vi "VFD_No TCHX.vi"() -> (0 "GS1 Communication Error Out":errorcluster)   [LabVIEW 2017]
uses:
  <vilib>/Platform/TimedLoop/XDataNode/timing_clust.ctl
  <vilib>/Platform/TimedLoop/XDataNode/nitl_modes.ctl
  <vilib>/Platform/TimedLoop/XDataNode/wakeup.ctl
  <vilib>/NI Modbus.llb/MB Serial Master Query Write Single Register (poly).vi
  <vilib>/Platform/TimedLoop/XDataNode/XDataNode.xnode
  <vilib>/Platform/TimedLoop/XDataNode/XDNodeRunTimeDep.lvlib
panel:
  in  "GS1 Communication Error In":errorcluster
  out "Iteration Duration":i64
  out "Finished Late? [i-1]":bool
  out "CTAH Initializaton Error":errorcluster
  out "CTAH Initialization Loop Time (ms)":u32
  out "Pump Initializaton Error":errorcluster
  out "Pump Initialization Loop Time (ms)":u32
  # "Troubleshooting Modbus communication using third-party VIs and native I/O Server"
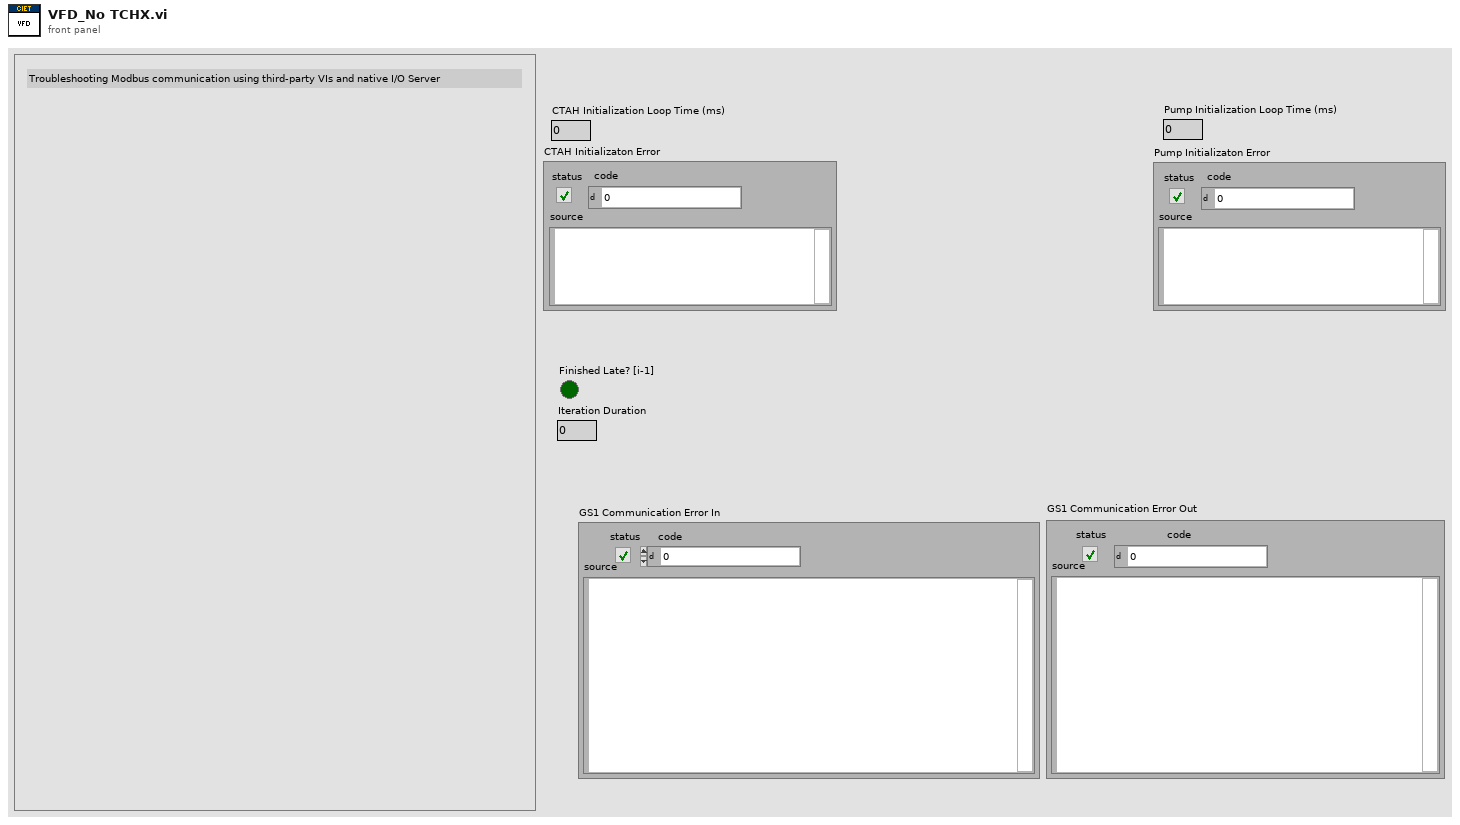
[diagram p1: front panel]
types:
  T1 = cluster{"Mode":enum16{"RTU", "ASCII"}, "Slave Address":u8}
  T2 = typedef "XDNodeRunTimeDep.lvlib/timing_clust.ctl" = cluster{"Expected End [f-1]":u64, "Actual End [f-1]":u64, "Finished Late? [f-1]":bool, "Expected End [i-1]":u64, "Actual End [i-1]":u64, "Finished Late? [i-1]":bool, "Expected Start [i]":u64, "Actual Start [i]":u64, "Expected Start [f]":u64, "Actual Start [f]":u64, "Source Name":string, "Structure Name":string, "Period":i64, "Deadline":i64, "Offset":i64, "Start":i64, "Priority":i32, "Timeout":i32, "Mode":T3, "Wakeup Reason":T4, "Error":errorcluster, "Source Type":string, "Secondary Source Type":string, "Global End Time":u64, "Global Start Time":u64, "Frame Duration":u64, "Iteration Duration":u64, "Assigned CPU":i32, "I/O Scan Engine Mode":u32}
  T3 = typedef "XDNodeRunTimeDep.lvlib/nitl_modes.ctl" = enum32{"No Change", "Process missed periods, maintain original phase", "Discard missed periods, maintain original phase", "Process missed periods, ignore original phase", "Discard missed periods, ignore original phase"}
  T4 = typedef "XDNodeRunTimeDep.lvlib/wakeup.ctl" = enum32{"Normal", "Aborted", "Asynchronous wakeup", "Timing source error", "Timed loop error", "Timeout"}
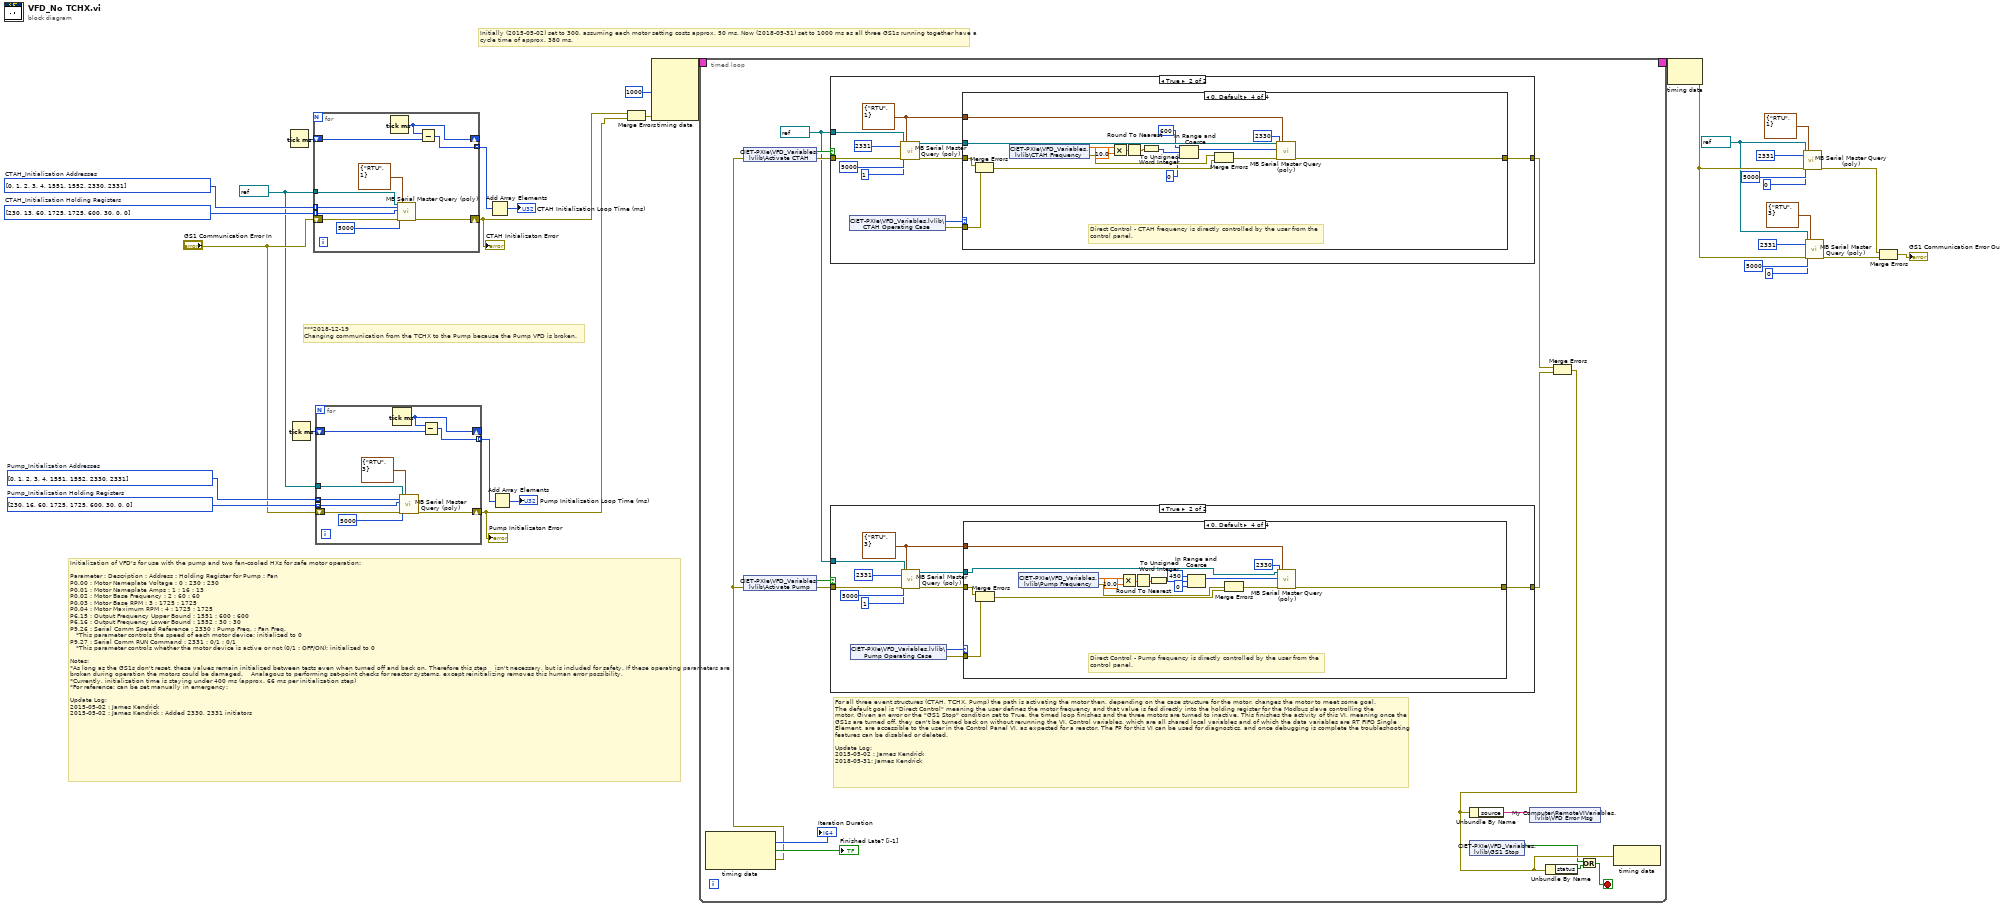
[diagram p0: block diagram]
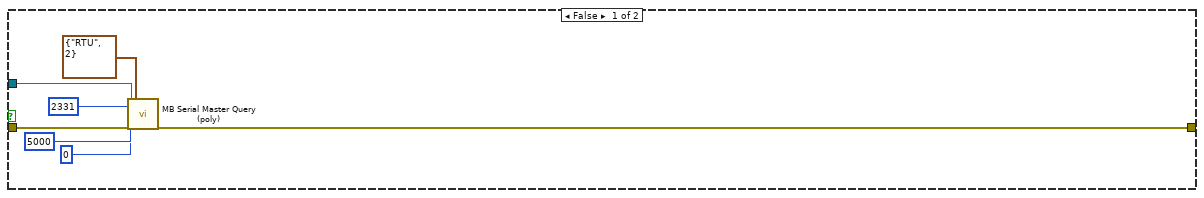
[diagram p2: hidden frame]
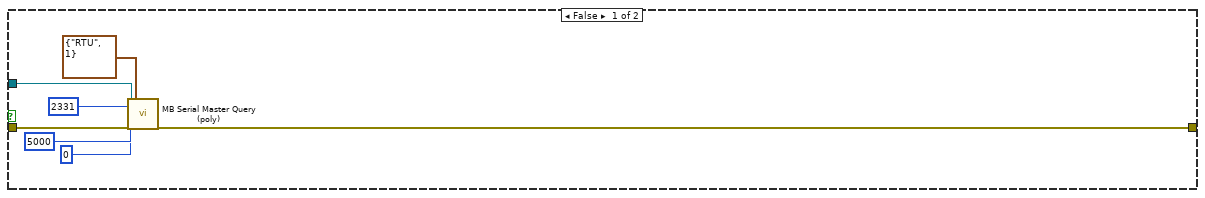
[diagram p6: hidden frame]
diagram:
  w4 = refnum<visa-resource-name> "VFD" ("VISA resource name")
  w5 = refnum<visa-resource-name> "VFD" ("VISA resource name")
  w22 = u16[] [230, 13, 60, 1725, 1725, 600, 30, 0, 0]  # CTAH_Initialization Holding Registers
  w23 = u16[] [0, 1, 2, 3, 4, 1551, 1552, 2330, 2331]  # CTAH_Initialization Addresses
  w30 = u16[] [230, 16, 60, 1725, 1725, 600, 30, 0, 0]  # Pump_Initialization Holding Registers
  w31 = u16[] [0, 1, 2, 3, 4, 1551, 1552, 2330, 2331]  # Pump_Initialization Addresses
  # "***2018-12-19\nChanging communication from the TCHX to the Pump because the Pump VFD is broken."
  # "Initially (2015-05-02) set to 300, assuming each motor setting costs approx. 50 ms. Now (2018-05-31) set to 1000 ms as all three GS1s running together have a \ncycle time of approx. 380 ms."
  # "Initialization of VFD's for use with the pump and two fan-cooled HXs for safe motor operation:\n\nParameter : Description : Address : Holding Register for Pump : Fan\nP0.00 : Motor Nameplate Voltage : 0 : 230 : 230\nP0.01 : Motor Nameplate Amps : 1 : 16 : 13\nP0.02 : Motor Base Frequency : 2 : 60 : 60\nP0.03 : Motor Base RPM : 3 : 1725 : 1725\nP0.04 : Motor Maximum RPM : 4 : 1725 : 1725\nP6.15 : Output Frequency Upper Bound : 1551 : 600 : 600\nP6.16 : Output Frequency Lower Bound : 1552 : 30 : 30\nP9.26 : Serial Comm Speed Reference : 2330 : Pump Freq. : Fan Freq. \n   *This parameter controls the speed of each motor device; initialized to 0\nP9.27 : Serial Comm RUN Command : 2331 : 0/1 : 0/1\n   *This parameter controls whether the motor device is active or not (0/1 : OFF/ON); initialized to 0\n\nNotes:\n*As long as the GS1s don't reset, these values remain initialized between tests even when turned off and back on. Therefore this step    isn't necessary, but is included for safety. If these operating parameters are broken during operation the motors could be damaged.    Analagous to performing set-point checks for reactor systems, except reinitializing removes this human error possibility.\n*Currently, initialization time is staying under 400 ms (approx. 66 ms per initialization step)\n*For reference; can be set manually in emergency:\n\nUpdate Log:\n2015-05-02 : James Kendrick \n2015-05-02 : James Kendrick : Added 2330, 2331 initiators"
  n1 = Tick Count (ms)() -> (millisecond timer value=w21:u32)
  n2 = Tick Count (ms)() -> (millisecond timer value=w29:u32)
  n3 = for {
    shift-right: [w39] -> w10
    shift-left: "GS1 Communication Error In" -> [w40]
    tunnel: w23 -> [w38] mode=indexing
    tunnel: w22 -> [w37] mode=indexing
    shift-right: [w34] -> _
    shift-left: w21 -> [w36]
    tunnel: [w35] -> w20 mode=indexing
    tunnel: w5 -> [w33]
    n4 = Tick Count (ms)() -> (millisecond timer value=w34:u32)
    n5 = call-poly <vilib>:"MB Serial Master Query (poly).vi"("VISA resource name"=w33, "Address"=w38, "Holding Register"=w37, "Timeout"=u32 5000, "error in"=w40, "Serial Parameters"=T1 {"Mode"=enum."RTU", "Slave Address"=1}) -> ("error out"=w39:errorcluster)  [unwired: 11 in, 2 out]
    n6 = Subtract(x=w34, y=w36) -> (x-y=w35:u32)
  }
  "CTAH Initializaton Error" <- w10
  n7 = for {
    shift-right: [w49] -> w1
    shift-left: "GS1 Communication Error In" -> [w50]
    tunnel: w31 -> [w48] mode=indexing
    tunnel: w30 -> [w47] mode=indexing
    shift-right: [w44] -> _
    shift-left: w29 -> [w46]
    tunnel: [w45] -> w28 mode=indexing
    tunnel: w5 -> [w43]
    n8 = Tick Count (ms)() -> (millisecond timer value=w44:u32)
    n9 = call-poly <vilib>:"MB Serial Master Query (poly).vi"("VISA resource name"=w43, "Address"=w48, "Holding Register"=w47, "Timeout"=u32 5000, "error in"=w50, "Serial Parameters"=T1 {"Mode"=enum."RTU", "Slave Address"=3}) -> ("error out"=w49:errorcluster)  [unwired: 11 in, 2 out]
    n10 = Subtract(x=w44, y=w46) -> (x-y=w45:u32)
  }
  "Pump Initializaton Error" <- w1
  n11 = Add Array Elements(numeric array=w20) -> (sum=→"CTAH Initialization Loop Time (ms)":u32)
  n12 = Add Array Elements(numeric array=w28) -> (sum=→"Pump Initialization Loop Time (ms)":u32)
  n13 = Merge Errors(w10, w1) -> (w12:errorcluster)
  n14 = node-c288(i64 1000 ("Pump Control Period (ms)"), w12) -> (w26:T2)  [unwired: 3 in]
  n15 = timed-loop {
    timing: w26 -> [_]
    timing-out: [_] -> w25
    stop <- w62 stop-if-true
    w56 = refnum<visa-resource-name> "VFD" ("VISA resource name")
    # "For all three event structures (CTAH, TCHX, Pump) the path is activating the motor then, depending on the case structure for the motor, changes the motor to meet some goal. \nThe default goal is \"Direct Control\" meaning the user defines the motor frequency and that value is fed directly into the holding register for the Modbus slave controlling the \nmotor. Given an error or the \"GS1 Stop\" condition set to True, the timed loop finishes and the three motors are turned to inactive. This finishes the activity of this VI, meaning once the\nGS1s are turned off, they can't be turned back on without rerunning the VI. Control variables, which are all shared local variables and of which the data variables are RT FIFO Single\nElement, are accessible to the user in the Control Panel VI, as expected for a reactor. The FP for this VI can be used for diagnostics, and once debugging is complete the troubleshooting\nfeatures can be disabled or deleted.  \n\nUpdate Log:\n2015-05-02 : James Kendrick\n2018-05-31: James Kendrick"
    n16 = node-c288() -> (→"Iteration Duration":i64, →"Finished Late? [i-1]":bool, w58:errorcluster)  [unwired: 1 in]
    n17 = shared-variable "CIET-PXIe\\VFD_Variables.lvlib\\Activate CTAH"(error in=w58) -> (w66:bool, error out=w65:errorcluster)
    n18 = shared-variable "CIET-PXIe\\VFD_Variables.lvlib\\Activate Pump"(error in=w58) -> (w61:bool, error out=w60:errorcluster)
    n19 = case shown="True" w66 {
      tunnel: w65 -> [w105 w115]
      tunnel: [w104 w111] -> w57
      tunnel: w56 -> [w103 w110]
      frame False {
        n20 = call-poly <vilib>:"MB Serial Master Query (poly).vi"("VISA resource name"=w103, "Address"=u16 2331, "Holding Register"=u16 0, "Timeout"=u32 5000, "error in"=w105, "Serial Parameters"=T1 {"Mode"=enum."RTU", "Slave Address"=1}) -> ("error out"=w104:errorcluster)  [unwired: 11 in, 2 out]
      }
      frame True {
        w109 = T1 {"Mode"=enum."RTU", "Slave Address"=1} ("Serial Parameters")
        n21 = shared-variable "CIET-PXIe\\VFD_Variables.lvlib\\CTAH Operating Case"() -> (w113:i32, error out=w112:errorcluster)  [unwired: 1 in]
        n22 = call-poly <vilib>:"MB Serial Master Query (poly).vi"("VISA resource name"=w110, "Address"=u16 2331, "Holding Register"=u16 1, "Timeout"=u32 5000, "error in"=w115, "Serial Parameters"=w109) -> ("VISA resource name out"=w114:refnum<visa-resource-name>, "error out"=w116:errorcluster)  [unwired: 11 in, 1 out]
        n23 = case shown="0, Default" w113 {
          tunnel: w116 -> [_ _ _ w135]
          tunnel: w114 -> [_ _ _ w136]
          tunnel: w112 -> [_ _ _ w134]
          tunnel: [_ _ _ w130] -> w111
          tunnel: w109 -> [_ _ _ w129]
          frame 1 {
            # "CTAH Outlet Temp: Feedback - CTAH frequency is determined by a\ncontrol function to hold the outlet temperature of the CTAH \nconstant."
          }
          frame 2 {
            # "Load Following - CTAH frequency is controlled to make the CTAH heat removal power\nto equal a user specified value through satisfying the equation: m_dot*c_P*(T_in - T_out)"
          }
          frame 3 {
            # "Dynamic Forcing - CTAH frequency is defined by a waveform function to drive the \nCTAH frequency and thus mass flow rate in a dynamic pattern, such as a square wave,\nsine wave, or other function as defined by the user.\n\nUser inputs to include:\nCTAH frequency set point (used as signal offset)\nSignal amplitude\nSignal frequency\nSignal type: sine, square, others?"
          }
          frame 0, Default {
            # "Direct Control - CTAH frequency is directly controlled by the user from the\ncontrol panel."
            n24 = Merge Errors(w135, w134) -> (w131:errorcluster)
            n25 = shared-variable "CIET-PXIe\\VFD_Variables.lvlib\\CTAH Frequency"() -> (w126:sgl, error out=w127:errorcluster)  [unwired: 1 in]
            n26 = Multiply(x=w126, y=sgl 10.0) -> (x*y=w128:sgl)
            n27 = Round To Nearest(number=w128) -> (nearest integer value=w125:sgl)
            n28 = To Unsigned Word Integer(number=w125) -> (unsigned 16bit integer=w123:u16)
            n29 = In Range and Coerce(upper limit=u16 600, x=w123, lower limit=u16 0) -> (coerced(x)=w122:u16)  [unwired: 1 out]
            n30 = Merge Errors(w127, w131) -> (w132:errorcluster)
            n31 = call-poly <vilib>:"MB Serial Master Query (poly).vi"("VISA resource name"=w136, "Address"=u16 2330, "Holding Register"=w122, "error in"=w132, "Serial Parameters"=w129) -> ("error out"=w130:errorcluster)  [unwired: 12 in, 2 out]
          }
        }
      }
    }
    n32 = case shown="True" w61 {
      tunnel: w60 -> [w70 w80]
      tunnel: [w69 w76] -> w53
      tunnel: w56 -> [w68 w75]
      frame False {
        n33 = call-poly <vilib>:"MB Serial Master Query (poly).vi"("VISA resource name"=w68, "Address"=u16 2331, "Holding Register"=u16 0, "Timeout"=u32 5000, "error in"=w70, "Serial Parameters"=T1 {"Mode"=enum."RTU", "Slave Address"=2}) -> ("error out"=w69:errorcluster)  [unwired: 11 in, 2 out]
      }
      frame True {
        w74 = T1 {"Mode"=enum."RTU", "Slave Address"=3} ("Serial Parameters")
        n34 = shared-variable "CIET-PXIe\\VFD_Variables.lvlib\\Pump Operating Case"() -> (w78:i32, error out=w77:errorcluster)  [unwired: 1 in]
        n35 = call-poly <vilib>:"MB Serial Master Query (poly).vi"("VISA resource name"=w75, "Address"=u16 2331, "Holding Register"=u16 1, "Timeout"=u32 5000, "error in"=w80, "Serial Parameters"=w74) -> ("VISA resource name out"=w79:refnum<visa-resource-name>, "error out"=w81:errorcluster)  [unwired: 11 in, 1 out]
        n36 = case shown="0, Default" w78 {
          tunnel: w81 -> [_ _ _ w101]
          tunnel: w79 -> [_ _ _ w91]
          tunnel: w77 -> [_ _ _ w100]
          tunnel: [_ _ _ w96] -> w76
          tunnel: w74 -> [_ _ _ w90]
          frame 1 {
            # "Mass Flow Rate: Feedback - Pump frequency is controlled through \na closed feedback to match a specified mass flow rate defined by \nthe user on the control panel."
          }
          frame 2 {
            # "Mass Flow Rate: Ramp - Pump frequency is controlled through a control function that\ncontrols the rate of change of the mass flow rate that the user specifies on the control\npanel to match a user desired final mass flow rate."
          }
          frame 3 {
            # "Dynamic Forcing - Pump frequency is defined by a waveform function to drive the \npump frequency and thus mass flow rate in a dynamic pattern, such as a square wave,\nsine wave, or other function as defined by the user.\n\nUser inputs to include:\nPump frequency set point (used as signal offset)\nSignal amplitude\nSignal frequency\nSignal type: sine, square, others?"
          }
          frame 0, Default {
            # "Direct Control - Pump frequency is directly controlled by the user from the\ncontrol panel."
            n37 = Merge Errors(w101, w100) -> (w97:errorcluster)
            n38 = shared-variable "CIET-PXIe\\VFD_Variables.lvlib\\Pump Frequency"() -> (w88:sgl, error out=w92:errorcluster)  [unwired: 1 in]
            n39 = Multiply(x=w88, y=sgl 10.0) -> (x*y=w89:sgl)
            n40 = Round To Nearest(number=w89) -> (nearest integer value=w86:sgl)
            n41 = To Unsigned Word Integer(number=w86) -> (unsigned 16bit integer=w85:u16)
            n42 = In Range and Coerce(upper limit=u16 450, x=w85, lower limit=u16 0) -> (coerced(x)=w93:u16)  [unwired: 1 out]
            n43 = Merge Errors(w92, w97) -> (w98:errorcluster)
            n44 = call-poly <vilib>:"MB Serial Master Query (poly).vi"("VISA resource name"=w91, "Address"=u16 2330, "Holding Register"=w93, "error in"=w98, "Serial Parameters"=w90) -> ("error out"=w96:errorcluster)  [unwired: 12 in, 2 out]
          }
        }
      }
    }
    n45 = shared-variable "CIET-PXIe\\VFD_Variables.lvlib\\GS1 Stop"() -> (w52:bool)  [unwired: 1 in, 1 out]
    n46 = Merge Errors(w57, w53) -> (w55:errorcluster)
    n47 = Unbundle By Name(w55) -> ("source"=w54:string)
    n48 = shared-variable "My Computer\\RemoteVIVariables.lvlib\\VFD Error Msg"(w54) -> ()  [unwired: 1 in, 1 out]
    n49 = Unbundle By Name(w55) -> ("status"=w59:bool)
    n50 = Or(x=w52, y=w59) -> (x .or. y?=w62:bool)
    n51 = node-c288(w55) -> ()  [unwired: 1 out]
  }
  n52 = node-c288(w25) -> (w6:errorcluster)
  n53 = call-poly <vilib>:"MB Serial Master Query (poly).vi"("VISA resource name"=w4, "Address"=u16 2331, "Holding Register"=u16 0, "Timeout"=u32 5000, "error in"=w6, "Serial Parameters"=T1 {"Mode"=enum."RTU", "Slave Address"=1}) -> ("error out"=w7:errorcluster)  [unwired: 11 in, 2 out]
  n54 = call-poly <vilib>:"MB Serial Master Query (poly).vi"("VISA resource name"=w4, "Address"=u16 2331, "Holding Register"=u16 0, "Timeout"=u32 5000, "error in"=w6, "Serial Parameters"=T1 {"Mode"=enum."RTU", "Slave Address"=3}) -> ("error out"=w8:errorcluster)  [unwired: 11 in, 2 out]
  n55 = Merge Errors(w7, w8) -> (→"GS1 Communication Error Out":errorcluster)
